vi "Burning Queue Init.vi"(8 "error in (no error) 2":errorcluster, 10 "Read:F/Wirte:T":bool, 11 "queue out":refnum<queue>) -> (0 "error out 2":errorcluster, 3 "queue out 2":refnum<queue>)   [LabVIEW 2022 SP3]
uses:
  Burning States.ctl
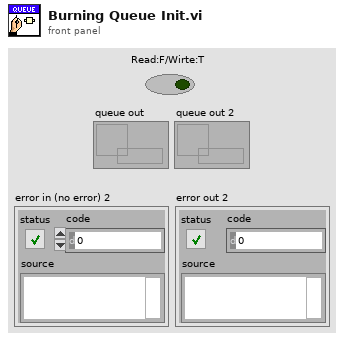
[diagram p1: front panel]
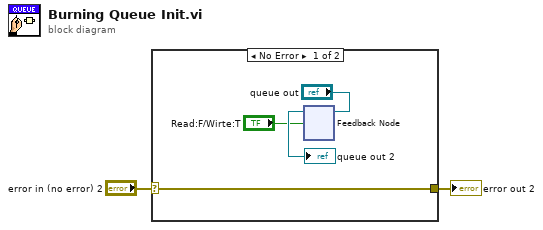
[diagram p0: block diagram]
diagram:
  n1 = case shown="No Error" "error in (no error) 2" {
    selector: "error in (no error) 2" -> [w6 w7]
    tunnel: [w6 w7] -> w1
    frame No Error {
      n2 = feedback-in #1("queue out", "Read:F/Wirte:T") -> ()
      n3 = feedback #1() -> (→"queue out 2":refnum<queue>)  [unwired: 1 in]
    }
    frame Error {
    }
  }
  "error out 2" <- w1
